vi "InitiateClientHandshake.vi"(6 "WS URI":string="ws://hostname.domain:80/resource/name", 7 "additional headers (none)":T1[](array[typedef]), 8 "error in (no error)":errorcluster, 9 "timeout ms (5000)":i32=5000, 10 "Relative URI Request (F)":bool, 11 "WebSocket Connection in":refnum<k5>) -> (0 "error out":errorcluster, 2 "Return Headers Out":variant, 3 "WebSocket Connection out":refnum<k5>)   [LabVIEW 2021, in "LV WebSockets.lvlib"]
doc: "Performs a client-side handshake. Sends the initial handshake HTTP header and waits for response from WebSocket server. Validates received accept key from the response.\nWebSockets 1.6.0.22\nSam Sharp - MediaMongrels Ltd\nCopyright (c) 2016, MediaMongrels Ltd"
uses:
  LV WebSockets.lvlib
  Headers.ctl
  Base64/Base64 Fast Encode 2012 NIVerified.vi
  <vilib>/ErrorRing/Error Ring.xnode
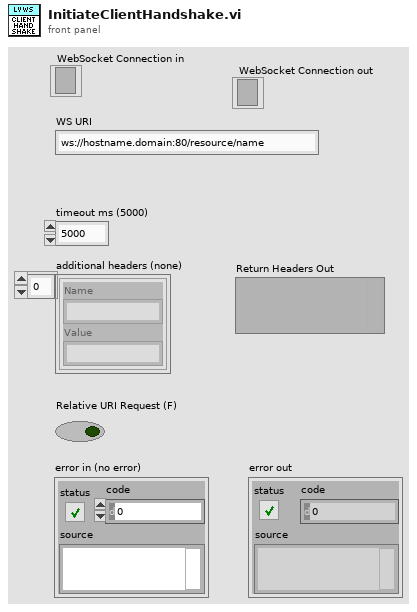
[diagram p1: front panel]
types:
  T1 = typedef "LV WebSockets.lvlib/Headers.ctl" = cluster{"Name":string, "Value":string}
  T2 = typedef "LV WebSockets.lvlib/HTTPResponseCodes.ctl" = u16
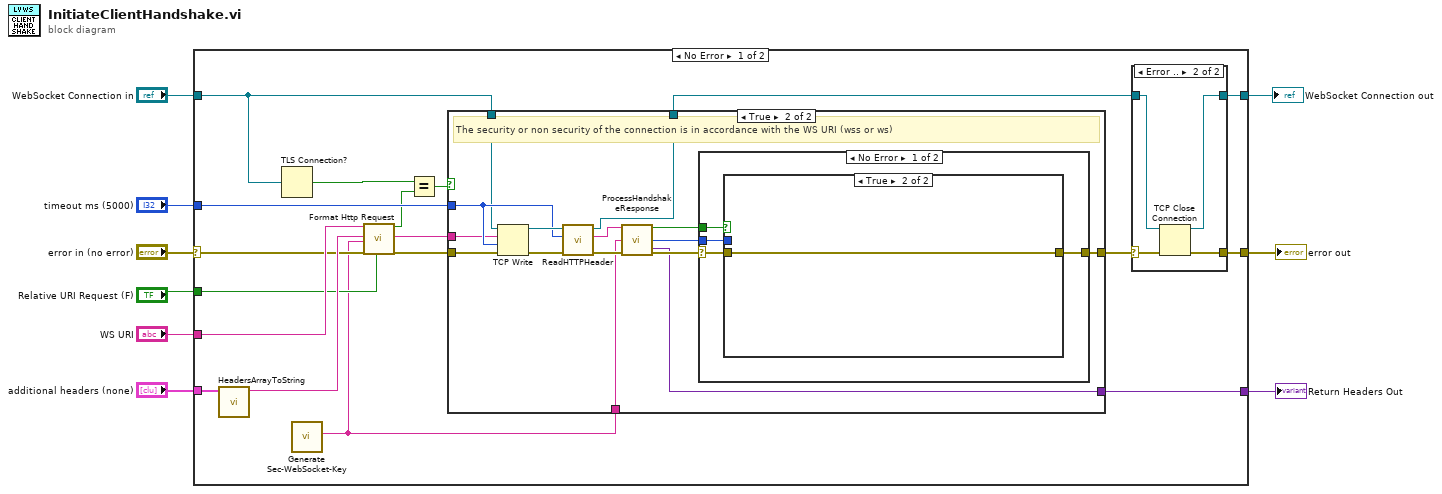
[diagram p0: block diagram]
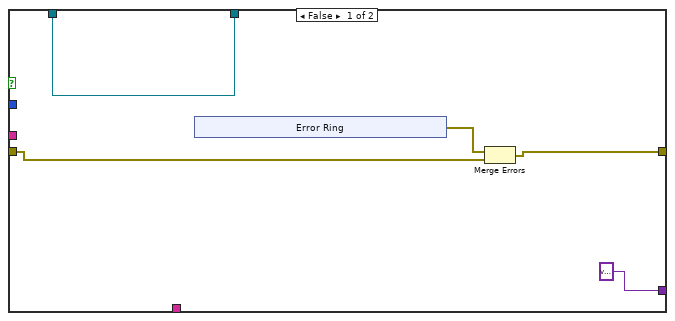
[diagram p3: hidden frame]
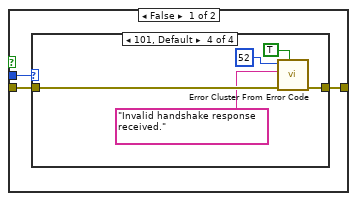
[diagram p4: hidden frame]
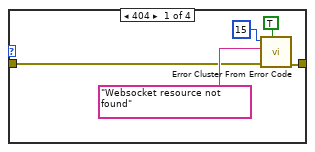
[diagram p5: hidden frame]
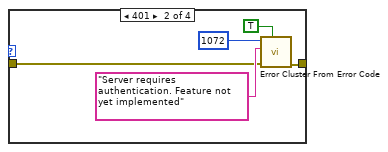
[diagram p6: hidden frame]
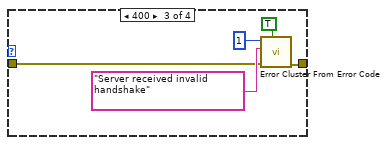
[diagram p7: hidden frame]
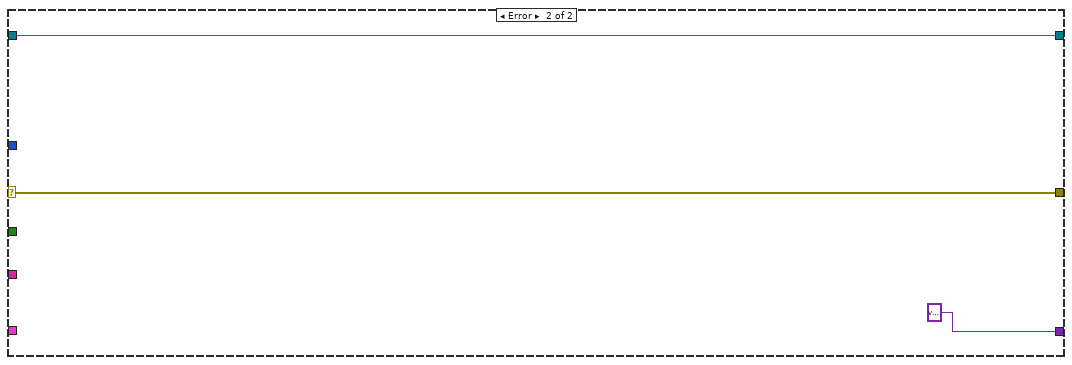
[diagram p9: hidden frame]
diagram:
  n1 = case shown="No Error" "error in (no error)" {
    selector: "error in (no error)" -> [w23 w90]
    tunnel: [w10 w89] -> w9
    tunnel: "WebSocket Connection in" -> [w17 w89]
    tunnel: [w12 w90] -> w6
    tunnel: "timeout ms (5000)" -> [w27 _]
    tunnel: [w18 variant ("Headers Out")] -> w4
    tunnel: "WS URI" -> [w24 _]
    tunnel: "additional headers (none)" -> [w26 _]
    tunnel: "Relative URI Request (F)" -> [w20 _]
    frame No Error {
      n2 = call "HeadersArrayToString.vi"("additional headers (none)"=w26) -> ("header string out"=w25:string)  [unwired: 10 in]
      n3 = TLS Connection?(1:w17) -> (0:w15:bool)
      n4 = call "Generate Sec-WebSocket-Key.vi"() -> ("Sec-WebSocket-Key"=w19:string)  [unwired: 11 in]
      n5 = call "Format Http Request.vi"("WS URI"=w24, "header string in"=w25, "WebSocket Key"=w19, "error in"=w23, "Relative URI Request (F)"=w20) -> ("Secure"=w16:bool, "Http Request"=w21:string, "error out"=w22:errorcluster)  [unwired: 12 in]
      n6 = Equal?(x=w15, y=w16) -> (x = y?=w14:bool)
      n7 = case shown="True" w14 {
        tunnel: w27 -> [_ w56]
        tunnel: [w37 w52] -> w11
        tunnel: [w38 w51] -> w13
        tunnel: w22 -> [w34 w50]
        tunnel: w21 -> [_ w49]
        tunnel: w19 -> [_ w47]
        tunnel: [variant ("Headers Out") w46] -> w18
        tunnel: w17 -> [w37 w44]
        frame False {
          n8 = xnode ("Error Ring")() -> ("error out"=w35:errorcluster)
          n9 = Merge Errors(w35, w34) -> (w38:errorcluster)
        }
        frame True {
          # "The security or non security of the connection is in accordance with the WS URI (wss or ws)"
          n10 = TCP Write(connection ID=w44, data in=w49, error in (no error)=w50, 9:w56) -> (connection ID out=w57:refnum<k5>, error out=w58:errorcluster)  [unwired: 1 out]
          n11 = call "ReadHTTPHeader.vi"("error in (no error)"=w58, "timeout ms (25000)"=w56, "WebSocket Connection in"=w57) -> ("error out"=w53:errorcluster, "HTTP Header"=w55:string, "WebSocket Connection out"=w52:refnum<k5>)  [unwired: 6 in]
          n12 = call "ProcessHandshakeResponse.vi"("HTTP Headers"=w55, "Sec-WebSocket-Key"=w47, "error in (no error)"=w53) -> ("Is Websocket Response?"=w48:bool, "Response Status Code"=w45:T2, "Headers Out"=w46:variant, "error out"=w54:errorcluster)  [unwired: 9 in]
          n13 = case shown="No Error" w54 {
            selector: w54 -> [w62 w87]
            tunnel: [w61 w87] -> w51
            tunnel: w48 -> [w60 _]
            tunnel: w45 -> [w59 _]
            frame No Error {
              n14 = case shown="True" w60 {
                tunnel: w62 -> [w64 w86]
                tunnel: [w65 w86] -> w61
                tunnel: w59 -> [w63 _]
                frame False {
                  n15 = case shown="101, Default" w63 {
                    tunnel: [w67 w72 w77 w85] -> w65
                    tunnel: w64 -> [w68 w73 w78 w84]
                    frame 404 {
                      n16 = call <vilib>:"Error Cluster From Error Code.vi"("show call chain? (False)"=TRUE, "error in (no error)"=w68, "error message (\"\")"="Websocket resource not found" ("error message (\"\")"), "error code (0)"=15) -> ("error out"=w67:errorcluster)  [unwired: 5 in]
                    }
                    frame 401 {
                      n17 = call <vilib>:"Error Cluster From Error Code.vi"("show call chain? (False)"=TRUE, "error in (no error)"=w73, "error message (\"\")"="Server requires authentication. Feature not yet implemented" ("error message (\"\")"), "error code (0)"=1072) -> ("error out"=w72:errorcluster)  [unwired: 5 in]
                    }
                    frame 400 {
                      n18 = call <vilib>:"Error Cluster From Error Code.vi"("show call chain? (False)"=TRUE, "error in (no error)"=w78, "error message (\"\")"="Server received invalid handshake" ("error message (\"\")"), "error code (0)"=1) -> ("error out"=w77:errorcluster)  [unwired: 5 in]
                    }
                    frame 101, Default {
                      n19 = call <vilib>:"Error Cluster From Error Code.vi"("show call chain? (False)"=TRUE, "error in (no error)"=w84, "error message (\"\")"="Invalid handshake response received." ("error message (\"\")"), "error code (0)"=52) -> ("error out"=w85:errorcluster)  [unwired: 5 in]
                    }
                  }
                }
                frame True {
                }
              }
            }
            frame Error {
            }
          }
        }
      }
      n20 = case shown="Error .." w13 {
        selector: w13 -> [w28 w33]
        tunnel: w11 -> [w29 w32]
        tunnel: [w29 w31] -> w10
        tunnel: [w28 w30] -> w12
        frame No Error {
        }
        frame Error {
          n21 = TCP Close Connection(connection ID=w32, error in (no error)=w33) -> (connection ID out=w31:refnum<k5>, error out=w30:errorcluster)  [unwired: 1 in]
        }
      }
    }
    frame Error {
    }
  }
  "WebSocket Connection out" <- w9
  "error out" <- w6
  "Return Headers Out" <- w4
